vi "ClosePanel.vi"(8 "error in (no error)":errorcluster, 11 "NI_DAQmx(AI) in":refnum<class "NI_DAQmx(AI).lvclass">) -> (0 "error out":errorcluster, 3 "NI_DAQmx(AI) out":refnum<class "NI_DAQmx(AI).lvclass">)   [LabVIEW 2025, in "NI_DAQmx(AI).lvclass"]
uses:
  NI_DAQmx(AI).lvclass
  NI_DAQmx(AI).lvclass/NI_DAQmx(AI).ctl
  DAQ_Abstr/Task_Type/AI_Task/AI_Task/AI_Task.lvclass
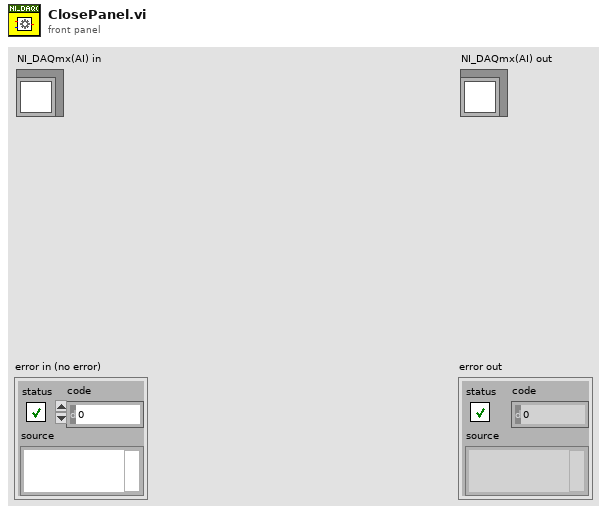
[diagram p1: front panel]
types:
  T1 = enum32{"Invalid", "Standard", "Closed", "Hidden", "Minimized", "Maximized"}
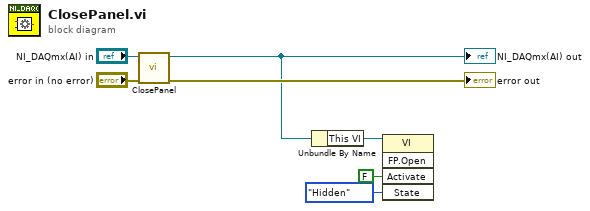
[diagram p0: block diagram]
diagram:
  n1 = call-parent "ClosePanel.vi"("error in (no error)"="error in (no error)", "Task_Abstr in"="NI_DAQmx(AI) in") -> ("error out"=→"error out":errorcluster, "Task_Abstr out"=w1:refnum<class "NI_DAQmx(AI).lvclass">)  [unwired: 8 in]
  "NI_DAQmx(AI) out" <- w1
  n2 = Unbundle By Name(w1) -> ("This VI"=w4:refnum<vi>)
  n3 = invoke class="VI" method="FP.Open"(reference=w4, "Activate"=FALSE ("Activate?"), "State"=T1."Hidden") -> ()  [unwired: 2 in, 5 out]
